vi "临时信号变比.vi"(9 "小信号变比":cluster{"UB":sgl, "IB":sgl, "UC":sgl}, 11 "串口号":refnum<visa-resource-name>) -> (10 "应答":string)   [LabVIEW 2014]
panel:
  out "完整帧":u8[](array[numeric]) format="%.0x"
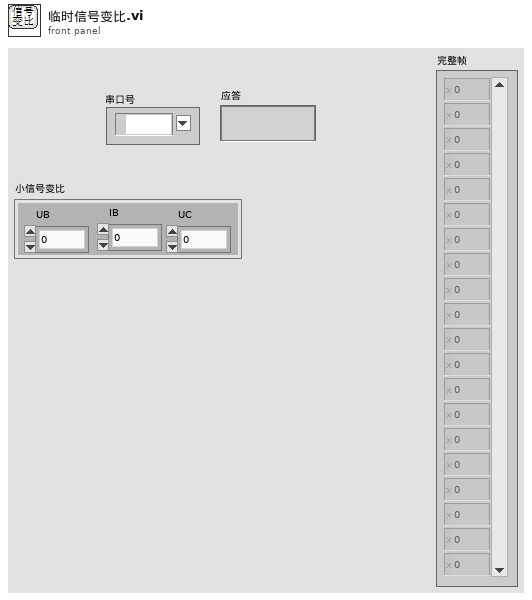
[diagram p1: front panel]
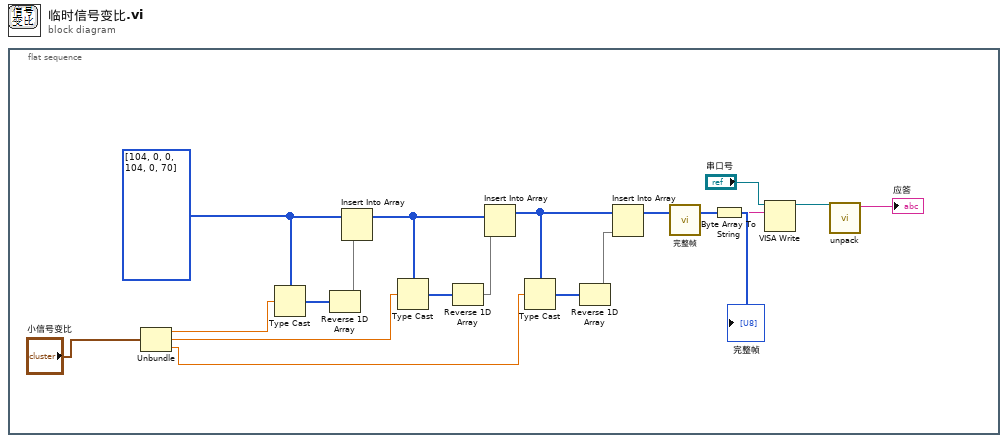
[diagram p0: block diagram]
diagram:
  n1 = flat-sequence {
    frame #0 {
      w12 = u8[] [104, 0, 0, 104, 0, 70]
      n2 = Unbundle("小信号变比") -> ("UB"=w3:sgl, "IB"=w2:sgl, "UC"=w1:sgl)
      n3 = Type Cast(type=w12, x=w3) -> (*(type *) &x=w13:u8[])
      n4 = Reverse 1D Array(array=w13) -> (reversed array=w11:u8[])
      n5 = Insert Into Array(array=w12, new element=w11) -> (w8:u8[])  [unwired: 1 in]
      n6 = Type Cast(type=w8, x=w2) -> (*(type *) &x=w10:u8[])
      n7 = Reverse 1D Array(array=w10) -> (reversed array=w7:u8[])
      n8 = Insert Into Array(array=w8, new element=w7) -> (w6:u8[])  [unwired: 1 in]
      n9 = Type Cast(type=w6, x=w1) -> (*(type *) &x=w9:u8[])
      n10 = Reverse 1D Array(array=w9) -> (reversed array=w5:u8[])
      n11 = Insert Into Array(array=w6, new element=w5) -> (w14:u8[])  [unwired: 1 in]
      n12 = call "完整帧.vi"("不完整帧"=w14) -> ("完整帧"=w19:u8[])  [unwired: 2 in]
      "完整帧" <- w19
      n13 = Byte Array To String(unsigned byte array=w19) -> (string=w18:string)
      n14 = VISA Write(VISA resource name="串口号", write buffer=w18) -> (VISA resource name out=w16:refnum<visa-resource-name>)  [unwired: 1 in, 2 out]
      n15 = call "unpack.vi"("串口号输入"=w16) -> ("应答"=→"应答":string)  [unwired: 5 in, 1 out]
    }
  }
